vi "temperature_read.vi"(8 "error in (no error)":errorcluster, 10 "Pin":u8 max=7 step=1, 11 "VISA resource name":refnum<visa-resource-name>) -> (0 "error out":errorcluster, 1 "Duty Cycle (%)":dbl, 2 "Temp threshold crossed":bool, 3 "VISA resource name out":refnum<visa-resource-name>)   [LabVIEW 2023]
uses:
  pico_scpi_labtool_labview_driver/scpi_driver/usbtmc_scpi_labtool.lvlib
panel:
  out "Temp Sensor":dbl
  # "Pin 0 - GP26\nPin 1 - GP28"
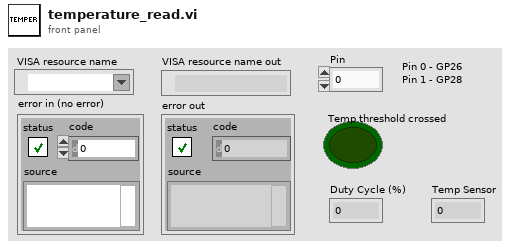
[diagram p1: front panel]
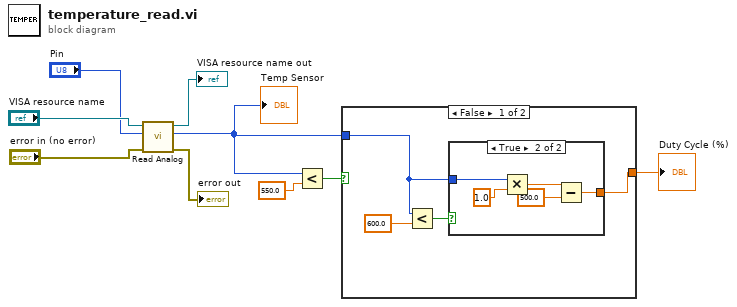
[diagram p0: block diagram]
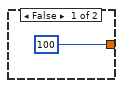
[diagram p2: hidden frame]
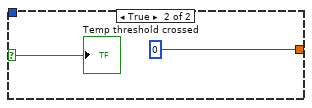
[diagram p3: hidden frame]
diagram:
  n1 = call "Read Analog.vi"("error in (no error)"="error in (no error)", "Pin"="Pin", "VISA resource name"="VISA resource name") -> ("error out"=→"error out":errorcluster, "analog out"=w1:i32, "VISA resource name out"=→"VISA resource name out":refnum<visa-resource-name>)  [unwired: 6 in]
  "Temp Sensor" <- w1
  n2 = Less?(x=w1, y=550.0) -> (x < y?=w3:bool)
  n3 = case shown="False" w3 {
    selector: w3 -> [_ w21]
    tunnel: [w11 0] -> w2
    tunnel: w1 -> [w10 _]
    frame False {
      n4 = Less?(x=w10, y=600.0) -> (x < y?=w13:bool)
      n5 = case shown="True" w13 {
        tunnel: [100 w17] -> w11
        tunnel: w10 -> [_ w15]
        frame False {
        }
        frame True {
          n6 = Multiply(x=w15, y=1.0 ("x")) -> (x*y=w19:dbl)
          n7 = Subtract(x=w19, y=500.0) -> (x-y=w17:dbl)
        }
      }
    }
    frame True {
      "Temp threshold crossed" <- w21
    }
  }
  "Duty Cycle (%)" <- w2
